vi "UMB_SampleActCommand.vi"(1 "act command":dbl[](array[numeric])) -> (0 "sampled act":dbl[](array[numeric]))   [LabVIEW 2012]
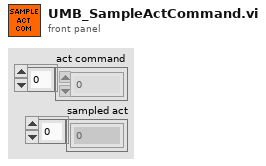
[diagram p1: front panel]
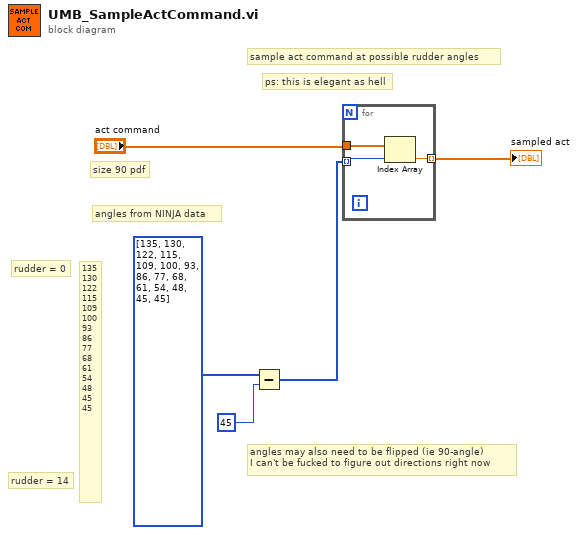
[diagram p0: block diagram]
diagram:
  # "rudder = 14"
  # "rudder = 0"
  # "angles may also need to be flipped (ie 90-angle)\nI can't be fucked to figure out directions right now"
  # "135\n130\n122\n115\n109\n100\n93\n86\n77\n68\n61\n54\n48\n45\n45"
  # "ps: this is elegant as hell"
  # "sample act command at possible rudder angles"
  # "angles from NINJA data"
  # "size 90 pdf"
  n1 = Subtract(x=i32[] [135, 130, 122, 115, 109, 100, 93, 86, 77, 68, 61, 54, 48, 45, 45] ("angles"), y=45) -> (x-y=w1:i32[])
  n2 = for {
    tunnel: "act command" -> [w8]
    tunnel: w1 -> [w7] mode=indexing
    tunnel: [w6] -> w4 mode=indexing
    n3 = Index Array(array=w8, index=w7) -> (element=w6:dbl)
  }
  "sampled act" <- w4
